vi "draw_tracking_image.vi"(8 "error in (no error)":errorcluster, 11 "Image In":T1) -> (0 "error out":errorcluster, 3 "Image Out":T1)   [LabVIEW 2019]
uses:
  <vilib>/vision/Image Controls.llb/IMAQ Image.ctl
  ActiveTracksFunctionalGlobalOperations.ctl
  ParametersGlobal.vi
  <vilib>/vision/NI_Vision_Development_Module.lvlib
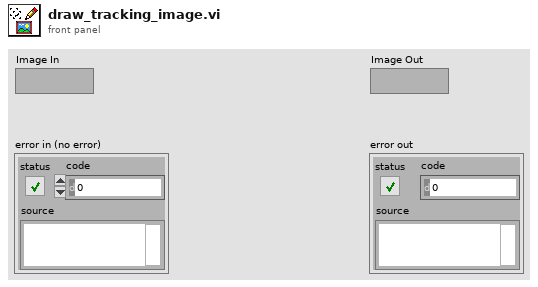
[diagram p1: front panel]
types:
  T1 = typedef "IMAQ Image.ctl" = refnum<image>
  T2 = typedef "ActiveTracksFunctionalGlobalOperations.ctl" = enum16{"Initialize", "ReadFullTrackGivenWormIndex", "WriteFullTrack", "ReadTrackSnippets", "WriteTrackGivenSnippets", "ReadStimulusSnippets", "StartNewTracksGivenSnippets", "EndTracksGivenSnippets", "WriteStimulusObjectGivenWormIndex", "CompleteAllActiveTracks", "ReturnAllActiveTrackIndecies"}
  T3 = typedef "WormTrackSnippetCluster.ctl" = cluster{"Track Centroid Positions (Camera Pixel)":sgl[][], "Within Track Index":i32, "Camera Buffer Indecies":i32[], "Area (Camera Pixels)":i32, "Speed (mm/s)":sgl, "Direction (radians)":sgl, "Centerline Positions (Camera Pixel)":sgl[][], "Ellipse Ratio":sgl, "Termination Reason":T4, "Track Index":i32, "Bounding Rect Left":i32, "Bounding Rect Top":i32, "Bounding Rect Right":i32, "Bounding Rect Bottom":i32, "Mature Camera Buffer":i32, "Start Camera Buffer Index":i32, "Reverse Started Camera Buffer":i32}
  T4 = typedef "TrackTerminationReasonEnum.ctl" = enum16{"StillActive", "MaxDisplacement", "NoBlobsLeft", "AreaIncrease", "AreaDecrease", "ExperimentEnded"}
  T5 = cluster{"Left":i32, "Top":i32, "Right":i32, "Bottom":i32}
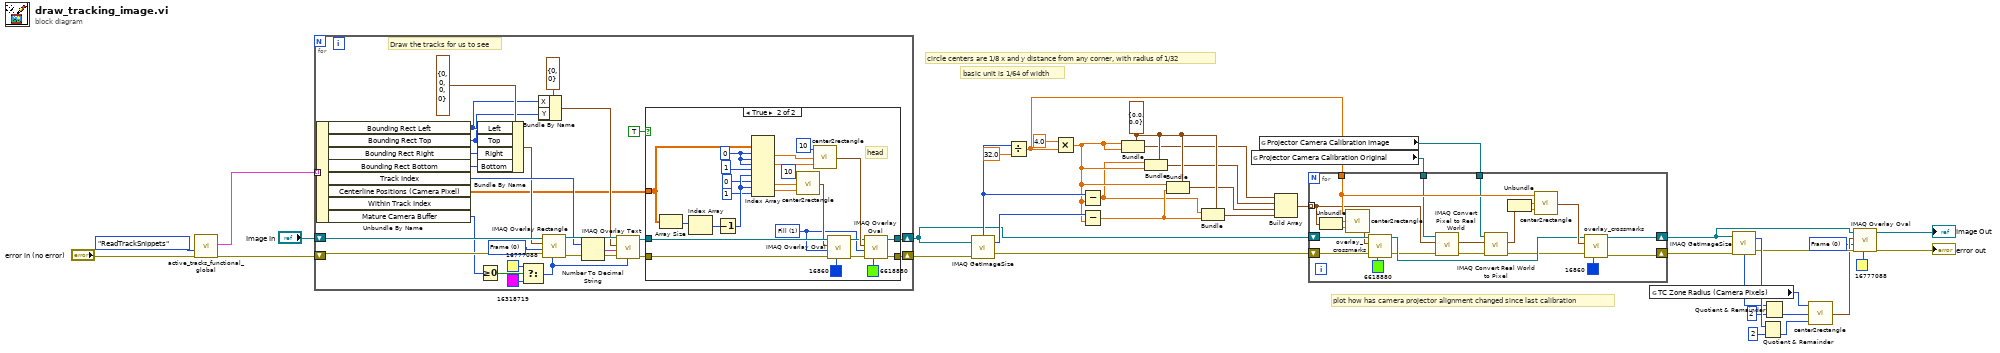
[diagram p0: block diagram]
diagram:
  w1 = u32 0 items=["Frame", "Fill"] ("Drawing Mode (Frame)")
  w26 = cluster{"X":sgl, "Y":sgl} {"X"=0.0, "Y"=0.0} ("Pixel Coordinates")
  # "plot how has camera projector alignment changed since last calibration"
  # "circle centers are 1/8 x and y distance from any corner, with radius of 1/32"
  # "basic unit is 1/64 of width"
  n1 = call "active_tracks_functional_global.vi"("error in"="error in (no error)", "Operations"=ActiveTracksFunctionalGlobalOperations."ReadTrackSnippets") -> ("error out"=w35:errorcluster, "Track Snippets Out"=w37:T3[])  [unwired: 5 in, 3 out]
  n2 = for {
    tunnel: w37 -> [w64] mode=indexing
    shift-right: [w47] -> w18
    shift-left: "Image In" -> [w65]
    shift-right: [w48] -> w34
    shift-left: w35 -> [w66]
    w63 = u32 0 items=["Frame", "Fill", "Highlight"] ("Drawing Mode (Frame)")
    # "Draw the tracks for us to see"
    n3 = Unbundle By Name(w64) -> ("Bounding Rect Left"=w52:i32, "Bounding Rect Top"=w51:i32, "Bounding Rect Right"=w55:i32, "Bounding Rect Bottom"=w54:i32, "Track Index"=w57:i32, "Centerline Positions (Camera Pixel)"=w45:sgl[][], "Mature Camera Buffer"=w44:i32)  [unwired: 1 out]
    n4 = Bundle By Name(cluster=T5 {"Left"=0, "Top"=0, "Right"=0, "Bottom"=0} ("Rectangle"), "Left"=w52, "Top"=w51, "Right"=w55, "Bottom"=w54) -> (w53:T5)
    n5 = Greater Or Equal To 0?(x=w44) -> (x >= 0?=w43:bool)
    n6 = Select(t=u32 16777088 ("Color"), s=w43, f=u32 16318719 ("Color")) -> (s? t:f=w40:u32)
    n7 = Bundle By Name(cluster=cluster{"X":i32, "Y":i32} {"X"=0, "Y"=0} ("Origin"), "X"=w52, "Y"=w51) -> (w59:cluster{"X":i32, "Y":i32})
    n8 = call "IMAQ Overlay Rectangle"("Color"=w40, "error in (no error)"=w66, "Drawing Mode (Frame)"=w63, "Rectangle"=w53, "Image"=w65) -> ("error out"=w61:errorcluster, "Image Out"=w62:T1)  [unwired: 5 in]
    n9 = Number To Decimal String(number=w57) -> (decimal integer string=w58:string)  [unwired: 1 in]
    n10 = call "IMAQ Overlay Text"("Text Color (black)"=w40, "error in (no error)"=w61, "String"=w58, "Origin"=w59, "Image"=w62) -> ("error out"=w50:errorcluster, "Image Out"=w49:T1)  [unwired: 5 in]
    n11 = case shown="True" TRUE {
      tunnel: w50 -> [w67 w91]
      tunnel: w49 -> [w68 w90]
      tunnel: [w67 w86] -> w48
      tunnel: [w68 w82] -> w47
      tunnel: w45 -> [_ w80]
      frame False {
      }
      frame True {
        w74 = 0 ("disabled index (col)")
        w81 = u32 1 items=["Frame", "Fill"] ("Drawing Mode (Frame)")
        # "head"
        n12 = Array Size(array=w80) -> (size(s)=w79:i32[])
        n13 = Index Array(array=w79) -> (element=w78:i32)  [unwired: 1 in]
        n14 = Decrement(x=w78) -> (x-1=w77:i32)
        n15 = Index Array(array=w80, index (row) #1=w74, index (col) #1=w74, index (row) #2=w74, index (col) #2=1 ("disabled index (col)"), index (row) #3=w77, index (col) #3=0 ("disabled index (col)"), index (row) #4=w77, index (col) #4=1 ("disabled index (col)")) -> (element #1=w72:sgl, element #2=w71:sgl, element #3=w70:sgl, element #4=w69:sgl)
        n16 = call "center2rectangle.vi"("Center Y"=w69, "Center X"=w70, "Box Half Size"=10) -> ("Box Rectangle"=w89:T5)
        n17 = call "center2rectangle.vi"("Center Y"=w71, "Center X"=w72, "Box Half Size"=10) -> ("Box Rectangle"=w84:T5)
        n18 = call "IMAQ Overlay Oval"("Color"=u32 16860, "error in (no error)"=w91, "Drawing Mode (Frame)"=w81, "Bounding Rectangle"=w89, "Image"=w90) -> ("error out"=w87:errorcluster, "Image Out"=w83:T1)  [unwired: 5 in]
        n19 = call "IMAQ Overlay Oval"("Color"=u32 6618880, "error in (no error)"=w87, "Drawing Mode (Frame)"=w81, "Bounding Rectangle"=w84, "Image"=w83) -> ("error out"=w86:errorcluster, "Image Out"=w82:T1)  [unwired: 5 in]
      }
    }
  }
  n20 = call "IMAQ GetImageSize"("Image"=w18, "error in (no error)"=w34) -> ("Y Resolution"=w30:i32, "X Resolution"=w31:i32, "error out"=w20:errorcluster)  [unwired: 2 in]
  n21 = Divide(x=w31, y=sgl 32.0) -> (x/y=w19:sgl)
  n22 = Multiply(x=sgl 4.0, y=w19) -> (x*y=w29:sgl)
  n23 = Subtract(x=w31, y=w29) -> (x-y=w27:sgl)
  n24 = Subtract(x=w30, y=w29) -> (x-y=w28:sgl)
  n25 = Bundle(cluster=w26, "X"=w29, "Y"=w29) -> (w22:cluster{"X":sgl, "Y":sgl})
  n26 = Bundle(cluster=w26, "X"=w27, "Y"=w29) -> (w23:cluster{"X":sgl, "Y":sgl})
  n27 = Bundle(cluster=w26, "X"=w29, "Y"=w28) -> (w24:cluster{"X":sgl, "Y":sgl})
  n28 = Bundle(cluster=w26, "X"=w27, "Y"=w28) -> (w25:cluster{"X":sgl, "Y":sgl})
  n29 = global read "ParametersGlobal.vi" "Projector Camera Calibration Original"() -> (w17:T1)
  n30 = global read "ParametersGlobal.vi" "Projector Camera Calibration Image"() -> (w16:T1)
  n31 = Build Array(w22, w23, w24, w25) -> (w21:cluster{"X":sgl, "Y":sgl}[])
  n32 = for {
    tunnel: w21 -> [w98] mode=indexing
    shift-right: [w105] -> w2
    shift-left: w18 -> [w114]
    shift-right: [w104] -> w11
    shift-left: w20 -> [w115]
    tunnel: w19 -> [w103]
    tunnel: w17 -> [w99]
    tunnel: w16 -> [w96]
    n33 = Unbundle(w98) -> ("X"=w112:sgl, "Y"=w111:sgl)
    n34 = call "center2rectangle.vi"("Center Y"=w111, "Center X"=w112, "Box Half Size"=w103) -> ("Box Rectangle"=w110:T5)
    n35 = call "overlay_crossmarks.vi"("Color"=u32 6618880, "error in (no error)"=w115, "Box Rectangle"=w110, "Refnum in"=w114) -> ("error out"=w102:errorcluster, "Refnum out"=w106:T1)  [unwired: 6 in]
    n36 = call "IMAQ Convert Pixel to Real World"("error in (no error)"=w102, "Pixel Coordinates"=w98, "Calibrated Image"=w99) -> ("error out"=w101:errorcluster, "Real World Coordinates"=w97:cluster{"X":sgl, "Y":sgl})  [unwired: 3 in, 4 out]
    n37 = call "IMAQ Convert Real World to Pixel"("error in (no error)"=w101, "Real World Coordinates"=w97, "Calibrated Image"=w96) -> ("error out"=w100:errorcluster, "Pixel Coordinates"=w95:cluster{"X":sgl, "Y":sgl})  [unwired: 3 in, 4 out]
    n38 = Unbundle(w95) -> ("X"=w109:sgl, "Y"=w108:sgl)
    n39 = call "center2rectangle.vi"("Center Y"=w108, "Center X"=w109, "Box Half Size"=w103) -> ("Box Rectangle"=w107:T5)
    n40 = call "overlay_crossmarks.vi"("Color"=u32 16860, "error in (no error)"=w100, "Box Rectangle"=w107, "Refnum in"=w106) -> ("error out"=w104:errorcluster, "Refnum out"=w105:T1)  [unwired: 6 in]
  }
  n41 = global read "ParametersGlobal.vi" "TC Zone Radius (Camera Pixels)"() -> (w4:i32)
  n42 = call "IMAQ GetImageSize"("Image"=w2, "error in (no error)"=w11) -> ("Y Resolution"=w14:i32, "X Resolution"=w12:i32, "error out"=w10:errorcluster)  [unwired: 2 in]
  n43 = Quotient & Remainder(x=w14, y=2) -> (floor(x/y)=w5:i32)  [unwired: 1 out]
  n44 = Quotient & Remainder(x=w12, y=2) -> (floor(x/y)=w6:i32)  [unwired: 1 out]
  n45 = call "center2rectangle.vi"("Center Y"=w5, "Center X"=w6, "Box Half Size"=w4) -> ("Box Rectangle"=w3:T5)
  n46 = call "IMAQ Overlay Oval"("Color"=u32 16777088, "error in (no error)"=w10, "Drawing Mode (Frame)"=w1, "Bounding Rectangle"=w3, "Image"=w2) -> ("error out"=→"error out":errorcluster, "Image Out"=→"Image Out":T1)  [unwired: 5 in]
